vi "gRPC Client Test.vi"() -> ()   [LabVIEW 2020, in "VeriStandgrpc_client.lvlib"]
uses:
  VeriStandgrpc_client.lvlib
  RPC Messages/veristand_Request.ctl
panel:
  in  "address":string="localhost:50051"
  out "error out":errorcluster
  in  "Stop":bool
  in  "Polling Rate (ms)":u32=100
  in  "Writer Channels":string[](array[string])=["Test", "Operator", "DUT", "Timestamp"]
  in  "New Data":string[](array[string])=["Dummy", "John123", "Golden", "5/1/2023"]
  out "Writer Status":string[](array[string])
  in  "Reader Channel":string[](array[string])=["Test", "Operator", "DUT", "Timestamp"]
  out "Data":string[](array[string])
  out "Reader Status":string[](array[string])
  out "Iteration":i32
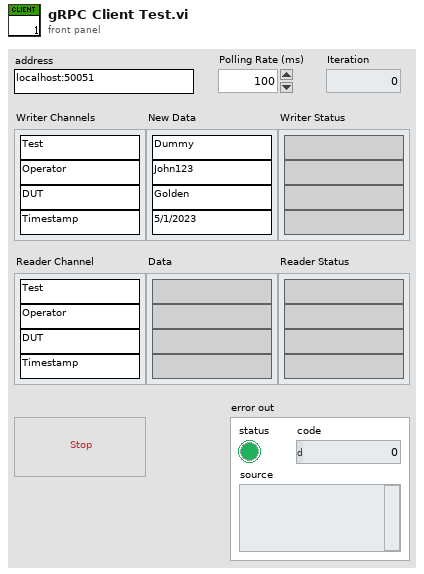
[diagram p1: front panel]
types:
  T1 = typedef "grpc-lvsupport-release.lvlib/grpcId.ctl" = u64
  T2 = typedef "VeriStandgrpc_client.lvlib/veristand_Request.ctl" = cluster{"server":string, "channel":string, "data":string}
  T3 = typedef "VeriStandgrpc_client.lvlib/veristand_Reponse.ctl" = cluster{"status":string, "data":string}
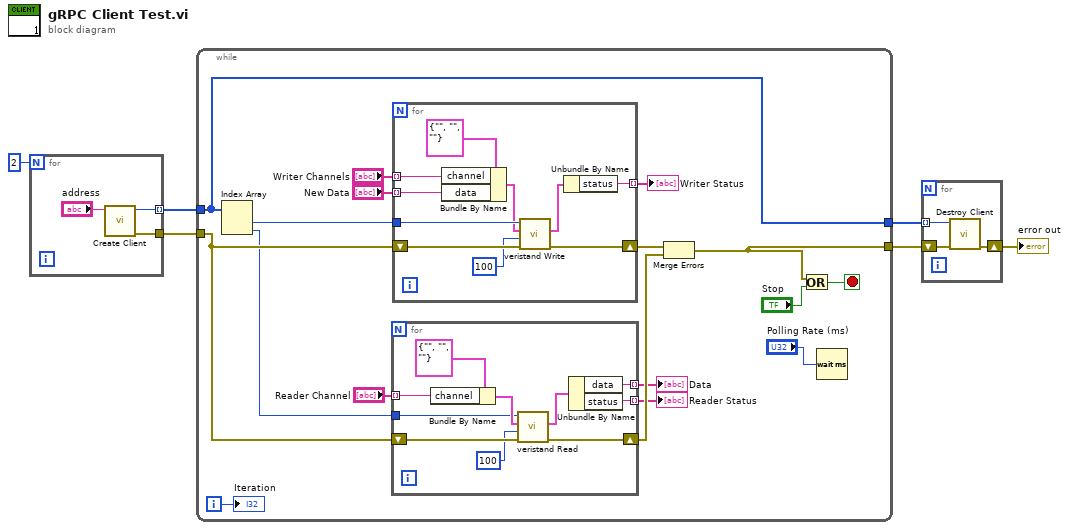
[diagram p0: block diagram]
diagram:
  n1 = for {
    N: 2 -> [_]
    tunnel: [w8] -> w6 mode=indexing
    tunnel: [w7] -> w5
    n2 = call "Create Client.vi"("address"="address") -> ("error out"=w7:errorcluster, "gRPC ID Out"=w8:T1)  [unwired: 9 in]
  }
  n3 = while {
    tunnel: w6 -> [w11]
    tunnel: w5 -> [w19]
    tunnel: [w11] -> w4
    tunnel: [w18] -> w3
    i -> [w10]
    stop <- w25 stop-if-true
    n4 = Index Array(array=w11) -> (element #1=w13:T1, element #2=w12:T1)  [unwired: 2 in]
    n5 = for {
      tunnel: "Reader Channel" -> [w35] mode=indexing
      tunnel: w12 -> [w33]
      shift-right: [w31] -> w17
      shift-left: w19 -> [w32]
      tunnel: [w29] -> w15 mode=indexing
      tunnel: [w28] -> w14 mode=indexing
      n6 = Bundle By Name(cluster=T2 {"server"="", "channel"="", "data"=""} ("Request Data"), "channel"=w35) -> (w34:T2)
      n7 = call "veristand Read.vi"("error in"=w32, "timeout (ms)"=100, "Request Data"=w34, "gRPC ID"=w33) -> ("error out"=w31:errorcluster, "Response Data"=w30:T3)  [unwired: 5 in, 1 out]
      n8 = Unbundle By Name(w30) -> ("data"=w29:string, "status"=w28:string)
    }
    "Data" <- w15
    "Reader Status" <- w14
    n9 = for {
      shift-right: [w44] -> w16
      shift-left: w19 -> [w45]
      tunnel: "Writer Channels" -> [w40] mode=indexing
      tunnel: "New Data" -> [w39] mode=indexing
      tunnel: [w38] -> w21 mode=indexing
      tunnel: w13 -> [w46]
      n10 = Bundle By Name(cluster=T2 {"server"="", "channel"="", "data"=""} ("Request Data"), "channel"=w40, "data"=w39) -> (w42:T2)
      n11 = call "veristand Write.vi"("error in"=w45, "timeout (ms)"=100, "Request Data"=w42, "gRPC ID"=w46) -> ("error out"=w44:errorcluster, "Response Data"=w41:T3)  [unwired: 5 in, 1 out]
      n12 = Unbundle By Name(w41) -> ("status"=w38:string)
    }
    "Writer Status" <- w21
    n13 = Merge Errors(w16, w17) -> (w18:errorcluster)
    n14 = Or(x=w18, y="Stop") -> (x .or. y?=w25:bool)
    n15 = Wait (ms)(milliseconds to wait="Polling Rate (ms)") -> ()  [unwired: 1 out]
    "Iteration" <- w10
  }
  n16 = for {
    tunnel: w4 -> [w49] mode=indexing
    shift-right: [w47] -> w2
    shift-left: w3 -> [w48]
    n17 = call "Destroy Client.vi"("error in"=w48, "gRPC ID"=w49) -> ("error out"=w47:errorcluster)  [unwired: 9 in]
  }
  "error out" <- w2
